vi "InsertFileFlowStep.vi"(8 "error in (no error)":errorcluster, 9 "add to beginning":bool, 10 "previous Fileflow step":string, 11 "new Fileflow step":string) -> (0 "error out":errorcluster)   [LabVIEW 2017, in "FileFlow.lvlib"]
doc: "Adds a process to a specific position within the Fileflow Script."
uses:
  <vilib>/addons/InsightCM/Devices/Shared/Common/FileFlow/FileFlow.lvlib
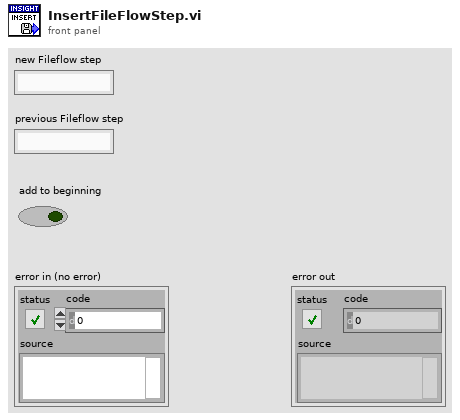
[diagram p1: front panel]
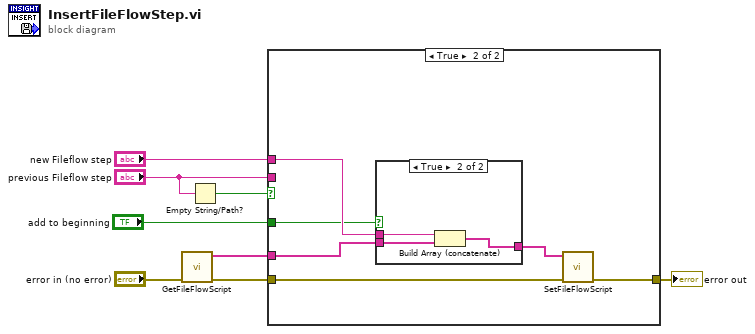
[diagram p0: block diagram]
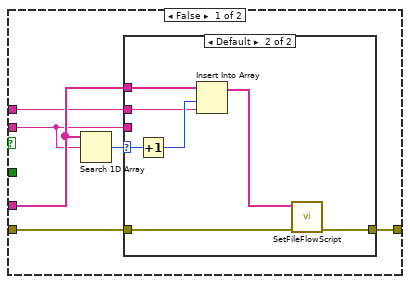
[diagram p2: hidden frame]
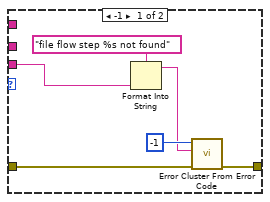
[diagram p3: hidden frame]
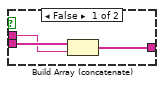
[diagram p4: hidden frame]
diagram:
  n1 = call <vilib>:"GetFileFlowScript.vi"("error in (no error)"="error in (no error)") -> ("error out"=w2:errorcluster, "Fileflow script"=w1:string[])  [unwired: 8 in, 1 out]
  n2 = Empty String/Path?(string/path="previous Fileflow step") -> (empty?=w5:bool)
  n3 = case shown="True" w5 {
    tunnel: w2 -> [w13 w29]
    tunnel: w1 -> [w12 w33]
    tunnel: [w11 w28] -> w8
    tunnel: "new Fileflow step" -> [w10 w32]
    tunnel: "previous Fileflow step" -> [w9 _]
    tunnel: "add to beginning" -> [_ w31]
    frame False {
      n4 = Search 1D Array(1D array=w12, element=w9) -> (index of element=w14:i32)  [unwired: 1 in]
      n5 = case shown="Default" w14 {
        selector: w14 -> [_ w24]
        tunnel: w12 -> [_ w27]
        tunnel: w10 -> [_ w25]
        tunnel: w13 -> [w20 w22]
        tunnel: [w19 w21] -> w11
        tunnel: w9 -> [w17 _]
        frame -1 {
          n6 = Format Into String(format string="file flow step %s not found", w17) -> (resulting string=w16:string)  [unwired: 2 in, 1 out]
          n7 = call <vilib>:"Error Cluster From Error Code.vi"("error in (no error)"=w20, "error message (\"\")"=w16, "error code (0)"=-1) -> ("error out"=w19:errorcluster)  [unwired: 6 in]
        }
        frame Default {
          n8 = Increment(x=w24) -> (x+1=w26:i32)
          n9 = Insert Into Array(array=w27, index=w26, new element=w25) -> (w23:string[])
          n10 = call <vilib>:"SetFileFlowScript.vi"("error in (no error)"=w22, "Fileflow script"=w23) -> ("error out"=w21:errorcluster)  [unwired: 9 in]
        }
      }
    }
    frame True {
      n11 = case shown="True" w31 {
        tunnel: w33 -> [w36 w39]
        tunnel: w32 -> [w35 w38]
        tunnel: [w34 w37] -> w30
        frame False {
          n12 = Build Array (concatenate)(w36, w35) -> (w34:string[])
        }
        frame True {
          n13 = Build Array (concatenate)(w38, w39) -> (w37:string[])
        }
      }
      n14 = call <vilib>:"SetFileFlowScript.vi"("error in (no error)"=w29, "Fileflow script"=w30) -> ("error out"=w28:errorcluster)  [unwired: 9 in]
    }
  }
  "error out" <- w8
